vi "FT_Write_FT2232_EEPROM.vi"(1 "FT2232 EEPROM Contents":T1={"Signature 1"=0, "Signature 2"=4294967295, "Version"=4, "Vendor ID"=1027, "Product ID"=24592, "Manufacturer"="FTDI", "Manufacturer ID"="FT", "Description"="", "Serial Number"="", "Max Power (mA)"=90, "PnP"=0, "Self Powered"=0, "Remote Wake-Up"=0, "Rev4"=0, "Iso In"=0, "Iso Out"=0, "Pull Down Enable"=0, "Serial Number Enable"=0, "USB Version Enable"=0, "USB Version"=512, "Rev5"=1, "Iso In A"=0, "Iso In B"=0, "Iso Out A"=0, "Iso Out B"=0, "Pull Down Enable"=0, "Serial Number Enable"=1, "USB Version Enable"=1, "USB Version"=512, "A Is High Current"=0, "B Is High Current"=0, "A Is 245 FIFO"=0, "A Is CPU FIFO"=0, "A Is Fast Serial"=0, "A Is VCP"=1, "B Is 245 FIFO"=0, "B Is CPU FIFO"=0, "B Is Fast Serial"=0, "B Is VCP"=1, "Use Ext Osc"=0, "High Drive IOs"=0, "Endpoint Size"=64, "Pull Down Enable R"=0, "Serial Number Enable R"=1, "Invert TXD"=0, "Invert RXD"=0, "Invert RTS"=0, "Invert CTS"=0, "Invert DTR"=0, "Invert DSR"=0, "Invert DCD"=0, "Invert RI"=0, "CBus0"=0, "CBus1"=0, "CBus2"=0, "CBus3"=0, "CBus4"=5, "R Is VCP"=0, "Pull Down Enable 7"=0, "Serial Number Enable 7"=0, "AL Slow Slew"=0, "AL Schmitt Input"=0, "AL Drive Current"=4, "AH Slow Slew"=0, "AH Schmitt Input"=0, "AH Drive Current"=4, "BL Slow Slew"=0, "BL Schmitt Input"=0, "BL Drive Current"=4, "BH Slow Slew"=0, "BH Schmitt Input"=0, "BH Drive Current"=4, "A Is 245 FIFO 7"=0, "A Is CPU FIFO 7"=0, "A Is Fast Serial 7"=0, "A Is VCP 7"=0, "B Is 245 FIFO 7"=0, "B Is CPU FIFO 7"=0, "B Is Fast Serial 7"=0, "B Is VCP 7"=0, "Power Save"=0, "Pull Down Enable 8"=0, "Serial Number Enable 8"=0, "A Slow Slew"=0, "A Schmitt Input"=0, "A Drive Current"=4, "B Slow Slew"=0, "B Schmitt Input"=0, "B Drive Current"=4, "C Slow Slew"=0, "C Schmitt Input"=0, "C Drive Current"=4, "D Slow Slew"=0, "D Schmitt Input"=0, "D Drive Current"=4, "A RI Is TXDEN"=0, "B RI Is TXDEN"=0, "C RI Is TXDEN"=0, "D RI Is TXDEN"=0, "A Is VCP 8"=0, "B Is VCP 8"=0, "C Is VCP8"=0, "D Is VCP 8"=0} {"D Is VCP 8" items=["D2XX", "VCP"]; "C Is VCP8" items=["D2XX", "VCP"]; "B Is VCP 8" items=["D2XX", "VCP"]; "A Is VCP 8" items=["D2XX", "VCP"]; "D RI Is TXDEN" items=["Disabled", "Enabled"]; "C RI Is TXDEN" items=["Disabled", "Enabled"]; "B RI Is TXDEN" items=["Disabled", "Enabled"]; "A RI Is TXDEN" items=["Disabled", "Enabled"]; "D Drive Current" items=["4mA"=4, "8mA"=8, "12mA"=12, "16mA"=16]; "D Schmitt Input" items=["Disabled", "Enabled"]; "D Slow Slew" items=["Disabled", "Enabled"]; "C Drive Current" items=["4mA"=4, "8mA"=8, "12mA"=12, "16mA"=16]; "C Schmitt Input" items=["Disabled", "Enabled"]; "C Slow Slew" items=["Disabled", "Enabled"]; "B Drive Current" items=["4mA"=4, "8mA"=8, "12mA"=12, "16mA"=16]; "B Schmitt Input" items=["Disabled", "Enabled"]; "B Slow Slew" items=["Disabled", "Enabled"]; "A Drive Current" items=["4mA"=4, "8mA"=8, "12mA"=12, "16mA"=16]; "A Schmitt Input" items=["Disabled", "Enabled"]; "A Slow Slew" items=["Disabled", "Enabled"]; "Serial Number Enable 8" items=["Disabled", "Enabled"]; "Pull Down Enable 8" items=["Disabled", "Enabled"]; "Power Save" items=["Disabled", "Enabled"]; "B Is VCP 7" items=["D2XX", "VCP"]; "B Is Fast Serial 7" items=["Disabled", "Enabled"]; "B Is CPU FIFO 7" items=["Disabled", "Enabled"]; "B Is 245 FIFO 7" items=["UART", "FIFO"]; "A Is VCP 7" items=["D2XX", "VCP"]; "A Is Fast Serial 7" items=["Disabled", "Enabled"]; "A Is CPU FIFO 7" items=["Disabled", "Enabled"]; "A Is 245 FIFO 7" items=["UART", "FIFO"]; "BH Drive Current" items=["4mA"=4, "8mA"=8, "12mA"=12, "16mA"=16]; "BH Schmitt Input" items=["Disabled", "Enabled"]; "BH Slow Slew" items=["Disabled", "Enabled"]; "BL Drive Current" items=["4mA"=4, "8mA"=8, "12mA"=12, "16mA"=16]; "BL Schmitt Input" items=["Disabled", "Enabled"]; "BL Slow Slew" items=["Disabled", "Enabled"]; "AH Drive Current" items=["4mA"=4, "8mA"=8, "12mA"=12, "16mA"=16]; "AH Schmitt Input" items=["Disabled", "Enabled"]; "AH Slow Slew" items=["Disabled", "Enabled"]; "AL Drive Current" items=["4mA"=4, "8mA"=8, "12mA"=12, "16mA"=16]; "AL Schmitt Input" items=["Disabled", "Enabled"]; "AL Slow Slew" items=["Disabled", "Enabled"]; "Serial Number Enable 7" items=["Disabled", "Enabled"]; "Pull Down Enable 7" items=["Disabled", "Enabled"]; "R Is VCP" items=["D2XX", "VCP"]; "CBus4" items=["TXDEN", "PWRON#", "TXLED#", "RXLED#", "TX & RXLED#", "SLEEP#", "48MHz Clock", "24MHz Clock", "12MHz Clock", "6MHz Clock"]; "CBus3" items=["TXDEN", "PWRON#", "TXLED#", "RXLED#", "TX & RXLED#", "SLEEP#", "48MHz Clock", "24MHz Clock", "12MHz Clock", "6MHz Clock", "IO Mode", "Bit-Bang WRn", "Bit-Bang RDn"]; "CBus2" items=["TXDEN", "PWRON#", "TXLED#", "RXLED#", "TX & RXLED#", "SLEEP#", "48MHz Clock", "24MHz Clock", "12MHz Clock", "6MHz Clock", "IO Mode", "Bit-Bang WRn", "Bit-Bang RDn"]; "CBus1" items=["TXDEN", "PWRON#", "TXLED#", "RXLED#", "TX & RXLED#", "SLEEP#", "48MHz Clock", "24MHz Clock", "12MHz Clock", "6MHz Clock", "IO Mode", "Bit-Bang WRn", "Bit-Bang RDn"]; "CBus0" items=["TXDEN", "PWRON#", "TXLED#", "RXLED#", "TX & RXLED#", "SLEEP#", "48MHz Clock", "24MHz Clock", "12MHz Clock", "6MHz Clock", "IO Mode", "Bit-Bang WRn", "Bit-Bang RDn"]; "Invert RI" items=["RI Not Inverted", "RI Inverted"]; "Invert DCD" items=["DCD Not Inverted", "DCD Inverted"]; "Invert DSR" items=["DSR Not Inverted", "DSR Inverted"]; "Invert DTR" items=["DTR Not Inverted", "DTR Inverted"]; "Invert CTS" items=["CTS Not Inverted", "CTS Inverted"]; "Invert RTS" items=["RTS Not Inverted", "RTS Inverted"]; "Invert RXD" items=["RXD Not Inverted", "RXD Inverted"]; "Invert TXD" items=["TXD Not Inverted", "TXD Inverted"]; "Serial Number Enable R" items=["Disabled", "Enabled"]; "Pull Down Enable R" items=["Disabled", "Enabled"]; "Endpoint Size" items=["64"=64, "32"=32, "16"=16, "8"=8, "4"=4]; "High Drive IOs" items=["Disabled", "Enabled"]; "Use Ext Osc" items=["Internal Oscillator", "External Oscillator"]; "B Is VCP" items=["D2XX", "VCP"]; "B Is Fast Serial" items=["Disabled", "Enabled"]; "B Is CPU FIFO" items=["Disabled", "Enabled"]; "B Is 245 FIFO" items=["UART", "FIFO"]; "A Is VCP" items=["D2XX", "VCP"]; "A Is Fast Serial" items=["Disabled", "Enabled"]; "A Is CPU FIFO" items=["Disabled", "Enabled"]; "A Is 245 FIFO" items=["UART", "FIFO"]; "B Is High Current" items=["Disabled", "Enabled"]; "A Is High Current" items=["Disabled", "Enabled"]; "USB Version" items=["USB 1.1"=272, "USB 2.0"=512]; "USB Version Enable" items=["Disabled", "Enabled"]; "Serial Number Enable" items=["Disabled", "Enabled"]; "Pull Down Enable" items=["Disabled", "Enabled"]; "Iso Out B" items=["Disabled", "Enabled"]; "Iso Out A" items=["Disabled", "Enabled"]; "Iso In B" items=["Disabled", "Enabled"]; "Iso In A" items=["Disabled", "Enabled"]; "USB Version" items=["USB 1.1"=272, "USB 2.0"=512]; "USB Version Enable" items=["Disabled", "Enabled"]; "Serial Number Enable" items=["Disabled", "Enabled"]; "Pull Down Enable" items=["Disabled", "Enabled"]; "Iso Out" items=["Disabled", "Enabled"]; "Iso In" items=["Disabled", "Enabled"]; "Remote Wake-Up" items=["Disabled", "Enabled"]; "Self Powered" items=["Bus Powered", "Self Powered"]; "PnP" items=["Disabled", "Enabled"]; "Product ID" format="%x"; "Vendor ID" format="%x"; "Signature 2" format="%x"}, 2 "Handle":u32) -> (0 "FT_Status":u32(ring) items=["FT_OK", "FT_INVALID_HANDLE", "FT_DEVICE_NOT_FOUND", "FT_DEVICE_NOT_OPENED", "FT_IO_ERROR", "FT_INSUFFICIENT_RESOURCES", "FT_INVALID_PARAMETER", "FT_INVALID_BAUD_RATE", "FT_DEVICE_NOT_OPENED_FOR_ERASE", "FT_DEVICE_NOT_OPENED_FOR_WRITE", "FT_FAILED_TO_WRITE_DEVICE", "FT_EEPROM_READ_FAILED", "FT_EEPROM_WRITE_FAILED", "FT_EEPROM_ERASE_FAILED", "FT_EEPROM_NOT_PRESENT", "FT_EEPROM_NOT_PROGRAMMED", "FT_INVALID_ARGS", "FT_NOT_SUPPORTED", "FT_OTHER_ERROR"])   [LabVIEW 2019, in "D2XX.lvlib"]
uses:
  D2XX.lvlib
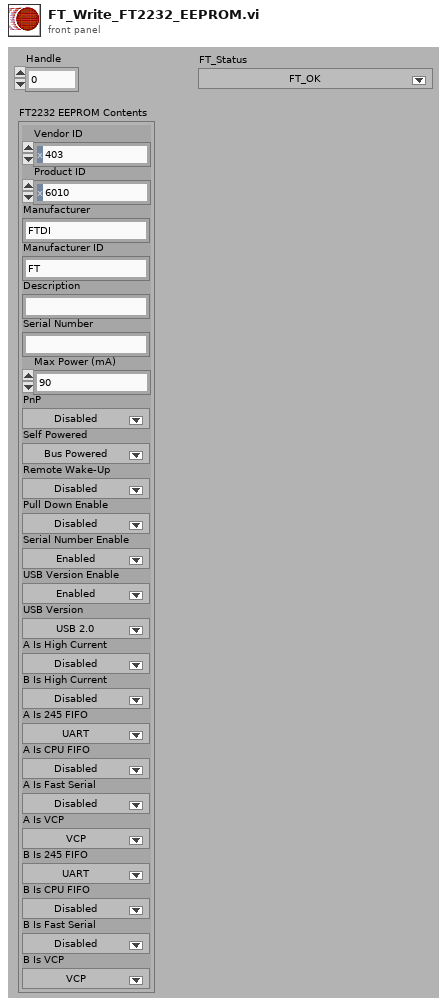
[diagram p1: front panel]
types:
  T1 = cluster{"Signature 1":u32, "Signature 2":u32, "Version":u32, "Vendor ID":u16, "Product ID":u16, "Manufacturer":string, "Manufacturer ID":string, "Description":string, "Serial Number":string, "Max Power (mA)":u16, "PnP":u16, "Self Powered":u16, "Remote Wake-Up":u16, "Rev4":u8, "Iso In":u8, "Iso Out":u8, "Pull Down Enable":u8, "Serial Number Enable":u8, "USB Version Enable":u8, "USB Version":u16, "Rev5":u8, "Iso In A":u8, "Iso In B":u8, "Iso Out A":u8, "Iso Out B":u8, "Pull Down Enable":u8, "Serial Number Enable":u8, "USB Version Enable":u8, "USB Version":u16, "A Is High Current":u8, "B Is High Current":u8, "A Is 245 FIFO":u8, "A Is CPU FIFO":u8, "A Is Fast Serial":u8, "A Is VCP":u8, "B Is 245 FIFO":u8, "B Is CPU FIFO":u8, "B Is Fast Serial":u8, "B Is VCP":u8, "Use Ext Osc":u8, "High Drive IOs":u8, "Endpoint Size":u8, "Pull Down Enable R":u8, "Serial Number Enable R":u8, "Invert TXD":u8, "Invert RXD":u8, "Invert RTS":u8, "Invert CTS":u8, "Invert DTR":u8, "Invert DSR":u8, "Invert DCD":u8, "Invert RI":u8, "CBus0":u8, "CBus1":u8, "CBus2":u8, "CBus3":u8, "CBus4":u8, "R Is VCP":u8, "Pull Down Enable 7":u8, "Serial Number Enable 7":u8, "AL Slow Slew":u8, "AL Schmitt Input":u8, "AL Drive Current":u8, "AH Slow Slew":u8, "AH Schmitt Input":u8, "AH Drive Current":u8, "BL Slow Slew":u8, "BL Schmitt Input":u8, "BL Drive Current":u8, "BH Slow Slew":u8, "BH Schmitt Input":u8, "BH Drive Current":u8, "A Is 245 FIFO 7":u8, "A Is CPU FIFO 7":u8, "A Is Fast Serial 7":u8, "A Is VCP 7":u8, "B Is 245 FIFO 7":u8, "B Is CPU FIFO 7":u8, "B Is Fast Serial 7":u8, "B Is VCP 7":u8, "Power Save":u8, "Pull Down Enable 8":u8, "Serial Number Enable 8":u8, "A Slow Slew":u8, "A Schmitt Input":u8, "A Drive Current":u8, "B Slow Slew":u8, "B Schmitt Input":u8, "B Drive Current":u8, "C Slow Slew":u8, "C Schmitt Input":u8, "C Drive Current":u8, "D Slow Slew":u8, "D Schmitt Input":u8, "D Drive Current":u8, "A RI Is TXDEN":u8, "B RI Is TXDEN":u8, "C RI Is TXDEN":u8, "D RI Is TXDEN":u8, "A Is VCP 8":u8, "B Is VCP 8":u8, "C Is VCP8":u8, "D Is VCP 8":u8}
  T2 = cluster{"Signature 1":u32, "Signature 2":u32, "Version":u32, "Vendor ID":u16, "Product ID":u16, u32, u32, u32, u32, "Max Power (mA)":u16, "PnP":u16, "Self Powered":u16, "Remote Wake-Up":u16, "Rev4":u8, "Iso In":u8, "Iso Out":u8, "Pull Down Enable":u8, "Serial Number Enable":u8, "USB Version Enable":u8, "USB Version":u16, "Rev5":u8, "Iso In A":u8, "Iso In B":u8, "Iso Out A":u8, "Iso Out B":u8, "Pull Down Enable":u8, "Serial Number Enable":u8, "USB Version Enable":u8, "USB Version":u16, "A Is High Current":u8, "B Is High Current":u8, "A Is 245 FIFO":u8, "A Is CPU FIFO":u8, "A Is Fast Serial":u8, "A Is VCP":u8, "B Is 245 FIFO":u8, "B Is CPU FIFO":u8, "B Is Fast Serial":u8, "B Is VCP":u8, "Use Ext Osc":u8, "High Drive IOs":u8, "Endpoint Size":u8, "Pull Down Enable R":u8, "Serial Number Enable R":u8, "Invert TXD":u8, "Invert RXD":u8, "Invert RTS":u8, "Invert CTS":u8, "Invert DTR":u8, "Invert DSR":u8, "Invert DCD":u8, "Invert RI":u8, "CBus0":u8, "CBus1":u8, "CBus2":u8, "CBus3":u8, "CBus4":u8, "R Is VCP":u8, "Pull Down Enable 7":u8, "Serial Number Enable 7":u8, "AL Slow Slew":u8, "AL Schmitt Input":u8, "AL Drive Current":u8, "AH Slow Slew":u8, "AH Schmitt Input":u8, "AH Drive Current":u8, "BL Slow Slew":u8, "BL Schmitt Input":u8, "BL Drive Current":u8, "BH Slow Slew":u8, "BH Schmitt Input":u8, "BH Drive Current":u8, "A Is 245 FIFO 7":u8, "A Is CPU FIFO 7":u8, "A Is Fast Serial 7":u8, "A Is VCP 7":u8, "B Is 245 FIFO 7":u8, "B Is CPU FIFO 7":u8, "B Is Fast Serial 7":u8, "B Is VCP 7":u8, "Power Save":u8, "Pull Down Enable 8":u8, "Serial Number Enable 8":u8, "A Slow Slew":u8, "A Schmitt Input":u8, "A Drive Current":u8, "B Slow Slew":u8, "B Schmitt Input":u8, "B Drive Current":u8, "C Slow Slew":u8, "C Schmitt Input":u8, "C Drive Current":u8, "D Slow Slew":u8, "D Schmitt Input":u8, "D Drive Current":u8, "A RI Is TXDEN":u8, "B RI Is TXDEN":u8, "C RI Is TXDEN":u8, "D RI Is TXDEN":u8, "A Is VCP 8":u8, "B Is VCP 8":u8, "C Is VCP8":u8, "D Is VCP 8":u8}
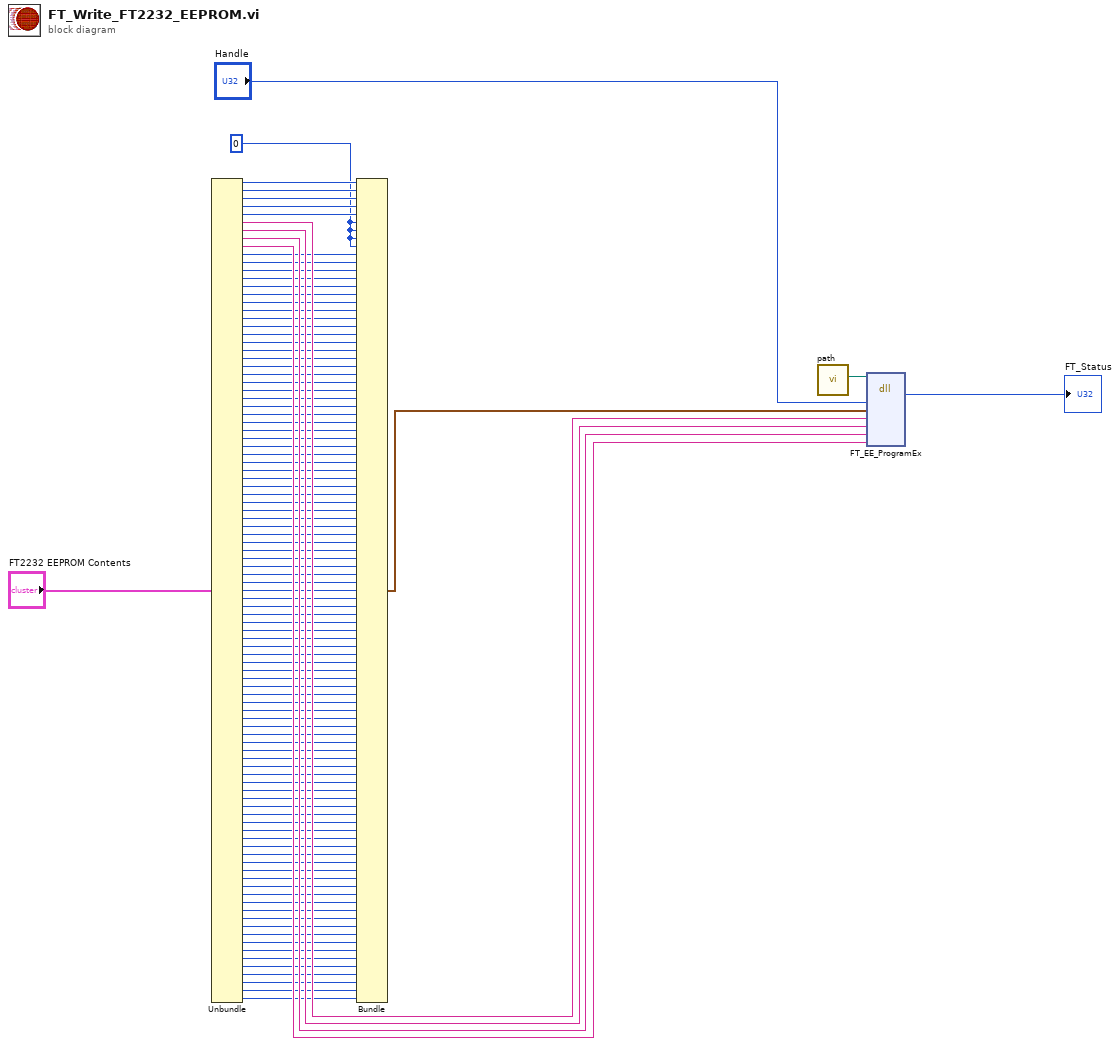
[diagram p0: block diagram]
diagram:
  w98 = u32 0
  n1 = Unbundle("FT2232 EEPROM Contents") -> ("Signature 1"=w103:u32, "Signature 2"=w102:u32, "Version"=w101:u32, "Vendor ID"=w100:u16, "Product ID"=w99:u16, "Manufacturer"=w107:string, "Manufacturer ID"=w106:string, "Description"=w105:string, "Serial Number"=w104:string, "Max Power (mA)"=w97:u16, "PnP"=w96:u16, "Self Powered"=w95:u16, "Remote Wake-Up"=w94:u16, "Rev4"=w93:u8, "Iso In"=w92:u8, "Iso Out"=w91:u8, "Pull Down Enable"=w90:u8, "Serial Number Enable"=w89:u8, "USB Version Enable"=w88:u8, "USB Version"=w87:u16, "Rev5"=w86:u8, "Iso In A"=w85:u8, "Iso In B"=w84:u8, "Iso Out A"=w83:u8, "Iso Out B"=w82:u8, "Pull Down Enable"=w81:u8, "Serial Number Enable"=w80:u8, "USB Version Enable"=w79:u8, "USB Version"=w77:u16, "A Is High Current"=w76:u8, "B Is High Current"=w75:u8, "A Is 245 FIFO"=w74:u8, "A Is CPU FIFO"=w73:u8, "A Is Fast Serial"=w72:u8, "A Is VCP"=w71:u8, "B Is 245 FIFO"=w70:u8, "B Is CPU FIFO"=w69:u8, "B Is Fast Serial"=w68:u8, "B Is VCP"=w67:u8, "Use Ext Osc"=w66:u8, "High Drive IOs"=w65:u8, "Endpoint Size"=w64:u8, "Pull Down Enable R"=w63:u8, "Serial Number Enable R"=w62:u8, "Invert TXD"=w61:u8, "Invert RXD"=w60:u8, "Invert RTS"=w59:u8, "Invert CTS"=w58:u8, "Invert DTR"=w57:u8, "Invert DSR"=w56:u8, "Invert DCD"=w55:u8, "Invert RI"=w53:u8, "CBus0"=w54:u8, "CBus1"=w52:u8, "CBus2"=w51:u8, "CBus3"=w50:u8, "CBus4"=w49:u8, "R Is VCP"=w48:u8, "Pull Down Enable 7"=w46:u8, "Serial Number Enable 7"=w45:u8, "AL Slow Slew"=w44:u8, "AL Schmitt Input"=w43:u8, "AL Drive Current"=w42:u8, "AH Slow Slew"=w41:u8, "AH Schmitt Input"=w40:u8, "AH Drive Current"=w39:u8, "BL Slow Slew"=w38:u8, "BL Schmitt Input"=w37:u8, "BL Drive Current"=w36:u8, "BH Slow Slew"=w35:u8, "BH Schmitt Input"=w34:u8, "BH Drive Current"=w33:u8, "A Is 245 FIFO 7"=w32:u8, "A Is CPU FIFO 7"=w31:u8, "A Is Fast Serial 7"=w30:u8, "A Is VCP 7"=w29:u8, "B Is 245 FIFO 7"=w28:u8, "B Is CPU FIFO 7"=w27:u8, "B Is Fast Serial 7"=w26:u8, "B Is VCP 7"=w24:u8, "Power Save"=w25:u8, "Pull Down Enable 8"=w23:u8, "Serial Number Enable 8"=w22:u8, "A Slow Slew"=w21:u8, "A Schmitt Input"=w20:u8, "A Drive Current"=w19:u8, "B Slow Slew"=w18:u8, "B Schmitt Input"=w17:u8, "B Drive Current"=w16:u8, "C Slow Slew"=w15:u8, "C Schmitt Input"=w14:u8, "C Drive Current"=w13:u8, "D Slow Slew"=w12:u8, "D Schmitt Input"=w11:u8, "D Drive Current"=w10:u8, "A RI Is TXDEN"=w9:u8, "B RI Is TXDEN"=w8:u8, "C RI Is TXDEN"=w7:u8, "D RI Is TXDEN"=w6:u8, "A Is VCP 8"=w5:u8, "B Is VCP 8"=w4:u8, "C Is VCP8"=w47:u8, "D Is VCP 8"=w2:u8)
  n2 = Bundle("Signature 1"=w103, "Signature 2"=w102, "Version"=w101, "Vendor ID"=w100, "Product ID"=w99, w98, w98, w98, w98, "Max Power (mA)"=w97, "PnP"=w96, "Self Powered"=w95, "Remote Wake-Up"=w94, "Rev4"=w93, "Iso In"=w92, "Iso Out"=w91, "Pull Down Enable"=w90, "Serial Number Enable"=w89, "USB Version Enable"=w88, "USB Version"=w87, "Rev5"=w86, "Iso In A"=w85, "Iso In B"=w84, "Iso Out A"=w83, "Iso Out B"=w82, "Pull Down Enable"=w81, "Serial Number Enable"=w80, "USB Version Enable"=w79, "USB Version"=w77, "A Is High Current"=w76, "B Is High Current"=w75, "A Is 245 FIFO"=w74, "A Is CPU FIFO"=w73, "A Is Fast Serial"=w72, "A Is VCP"=w71, "B Is 245 FIFO"=w70, "B Is CPU FIFO"=w69, "B Is Fast Serial"=w68, "B Is VCP"=w67, "Use Ext Osc"=w66, "High Drive IOs"=w65, "Endpoint Size"=w64, "Pull Down Enable R"=w63, "Serial Number Enable R"=w62, "Invert TXD"=w61, "Invert RXD"=w60, "Invert RTS"=w59, "Invert CTS"=w58, "Invert DTR"=w57, "Invert DSR"=w56, "Invert DCD"=w55, "Invert RI"=w53, "CBus0"=w54, "CBus1"=w52, "CBus2"=w51, "CBus3"=w50, "CBus4"=w49, "R Is VCP"=w48, "Pull Down Enable 7"=w46, "Serial Number Enable 7"=w45, "AL Slow Slew"=w44, "AL Schmitt Input"=w43, "AL Drive Current"=w42, "AH Slow Slew"=w41, "AH Schmitt Input"=w40, "AH Drive Current"=w39, "BL Slow Slew"=w38, "BL Schmitt Input"=w37, "BL Drive Current"=w36, "BH Slow Slew"=w35, "BH Schmitt Input"=w34, "BH Drive Current"=w33, "A Is 245 FIFO 7"=w32, "A Is CPU FIFO 7"=w31, "A Is Fast Serial 7"=w30, "A Is VCP 7"=w29, "B Is 245 FIFO 7"=w28, "B Is CPU FIFO 7"=w27, "B Is Fast Serial 7"=w26, "B Is VCP 7"=w24, "Power Save"=w25, "Pull Down Enable 8"=w23, "Serial Number Enable 8"=w22, "A Slow Slew"=w21, "A Schmitt Input"=w20, "A Drive Current"=w19, "B Slow Slew"=w18, "B Schmitt Input"=w17, "B Drive Current"=w16, "C Slow Slew"=w15, "C Schmitt Input"=w14, "C Drive Current"=w13, "D Slow Slew"=w12, "D Schmitt Input"=w11, "D Drive Current"=w10, "A RI Is TXDEN"=w9, "B RI Is TXDEN"=w8, "C RI Is TXDEN"=w7, "D RI Is TXDEN"=w6, "A Is VCP 8"=w5, "B Is VCP 8"=w4, "C Is VCP8"=w47, "D Is VCP 8"=w2) -> (w78:T2)  [unwired: 1 in]
  n3 = call "path.vi"() -> ("lib path"=w1:path)
  n4 = dll-call lib="FTD2XX.dll" fn="FT_EE_ProgramEx" label="FT_EE_WriteEx"(path in=w1, "Handle"="Handle", "FT_Program_Data"=w78, "Manufacturer"=w107, "Manufacturer ID"=w106, "Description"=w105, "Serial Number"=w104) -> (→"FT_Status":u32)  [unwired: 8 in, 2 out]
